vi "Write Variant Data.vi"(8 "error in (no error)":errorcluster, 10 "data":variant, 11 "Base Interface in":refnum<class "Base Interface.lvclass">) -> (0 "error out":errorcluster, 3 "Base Interface out":refnum<class "Base Interface.lvclass">)   [LabVIEW 2020, in "PV Access.lvlib" / "PV Data.lvlib" / "Base Interface.lvclass"]
uses:
  Base Interface.lvclass
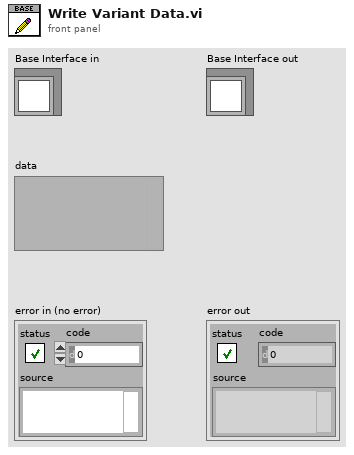
[diagram p1: front panel]
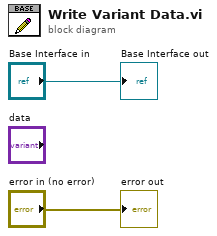
[diagram p0: block diagram]
diagram:
  "error out" <- "error in (no error)"
  "Base Interface out" <- "Base Interface in"
